vi "总氮流程.vi"   [LabVIEW 2016]
types:
  T1 = enum16{"步骤1", "步骤2", "步骤3", "步骤4", "步骤5", "步骤6", "步骤7", "步骤8", "步骤9", "步骤10"}
  T2 = enum32{"Bad", "Idle", "Run top level", "Running"}
  T3 = cluster{"系统时间":timestamp, "工作状态":u16, "测量模式":u16, "告警代码":enum16{"无告警", "缺试剂告警", "缺水样告警", "缺蒸馏水告警", "缺标液告警", "仪表漏液告警", "标定异常告警", "超量程告警", "加热异常", "低试剂预警", "超上限告警", "超下限告警", "仪表内部其他异常", "滴定异常告警", "电极异常告警", "量程切换告警", "参数设置告警", "PH电极电位异常", "电导率电极异常", "浊度光度异常", "溶解氧电极异常", "溶解氧光强异常", "温度异常告警", "PH异常告警", "溶解氧异常告警", "电导率异常告警", "浊度异常告警", "叶绿素异常告警", "藻密度异常告警", "蓝绿藻异常告警", "ORP异常告警", "氨氮异常告警", "清洁刷异常告警", "SD卡异常告警", "蓝牙异常告警", "Wifi异常告警", "流程异常告警"}, "故障代码":enum16{"无故障", "电机故障", "温度故障", "通讯故障", "滴定故障"}, "日志代码":u16, "软件版本":u16, "F0":sgl, "F1":sgl, "F2":sgl, "F3":sgl, "T":sgl, "H":sgl, "id":u16, "flowid":u16, "量程":u16}
  T4 = cluster{"因子编码":u32, "单位":u16, "标样参考值":sgl, "水样数据时间":timestamp, "水样实测值":sgl, "水样数据标识":string, "标样数据时间":timestamp, "标样实测值":sgl, "标样数据标识":string, "空白数据时间":timestamp, "空白实测值":sgl, "空白数据标识":string, "零点核查数据时间":timestamp, "零点核查实测值":sgl, "零点核查数据标识":string, "跨度核查数据时间":timestamp, "跨度核查实测值":sgl, "跨度核查数据标识":string, "加标回收数据时间":timestamp, "加标回收实测值":sgl, "加标回收数据标识":string, "平行样数据时间":timestamp, "平行样实测值":sgl, "平行样数据标识":string}
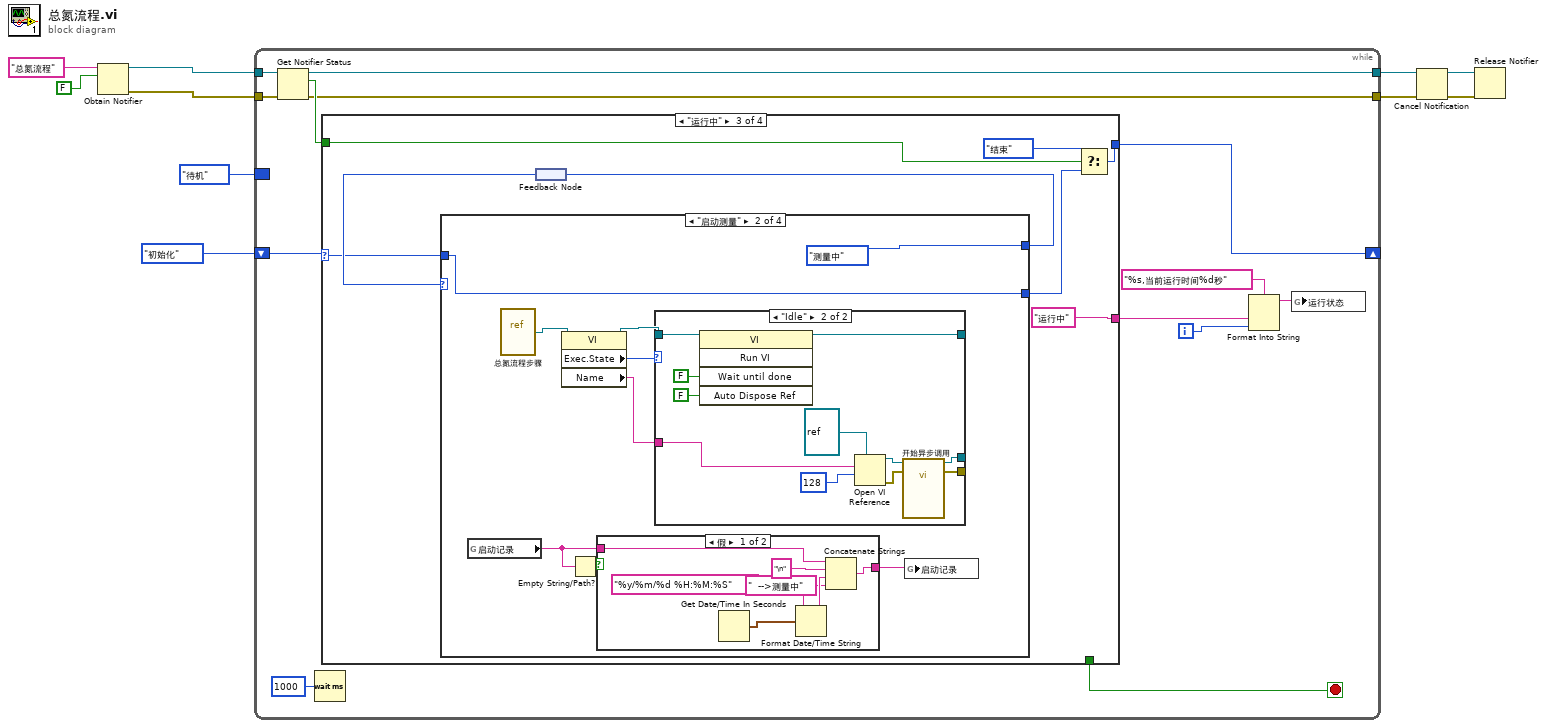
[diagram p0: block diagram]
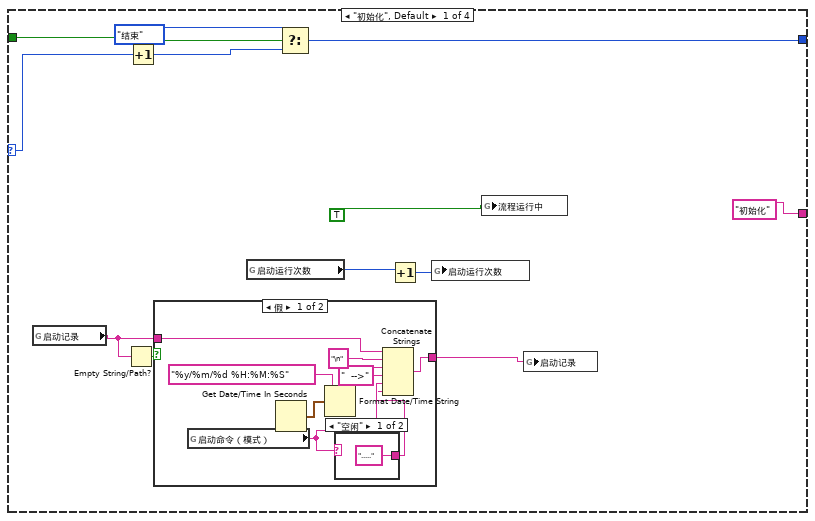
[diagram p2: hidden frame]
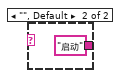
[diagram p3: hidden frame]
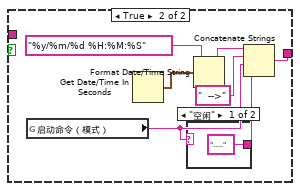
[diagram p4: hidden frame]
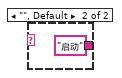
[diagram p5: hidden frame]
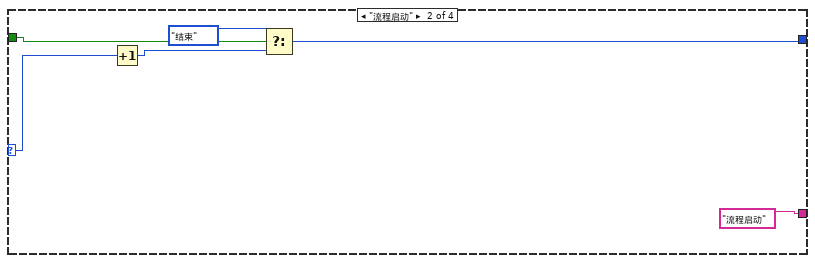
[diagram p6: hidden frame]
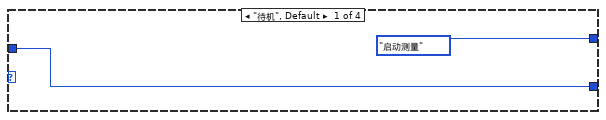
[diagram p7: hidden frame]
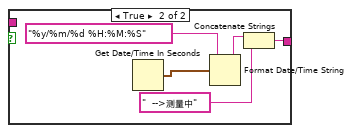
[diagram p8: hidden frame]
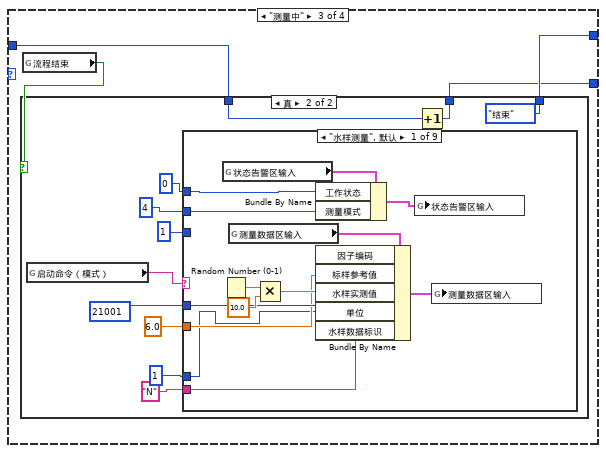
[diagram p10: hidden frame]
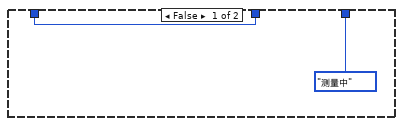
[diagram p11: hidden frame]
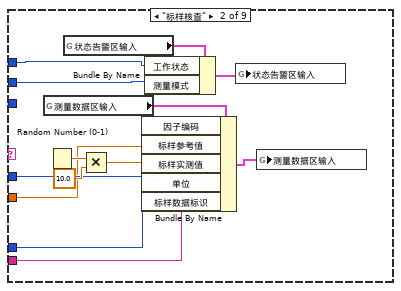
[diagram p12: hidden frame]
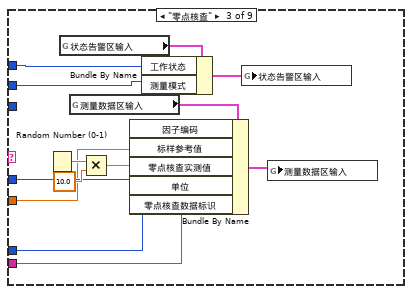
[diagram p13: hidden frame]
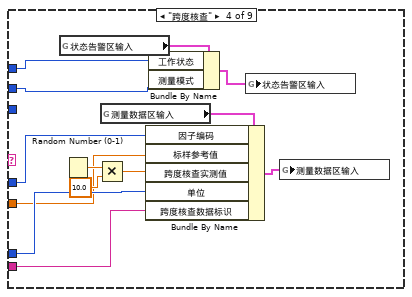
[diagram p14: hidden frame]
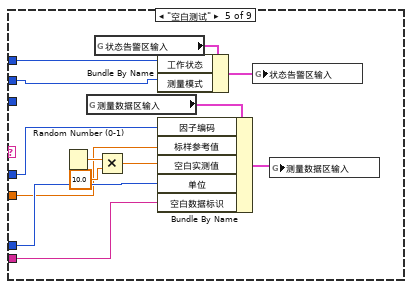
[diagram p15: hidden frame]
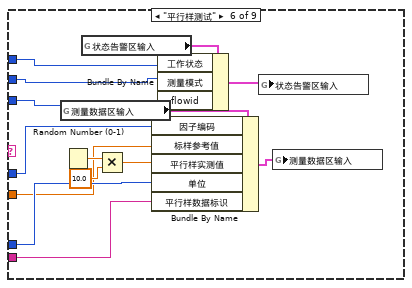
[diagram p16: hidden frame]
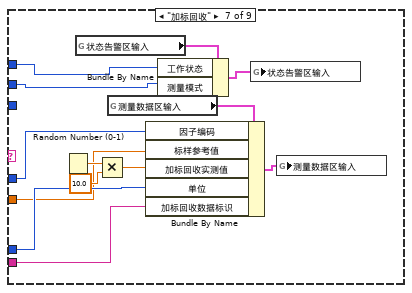
[diagram p17: hidden frame]
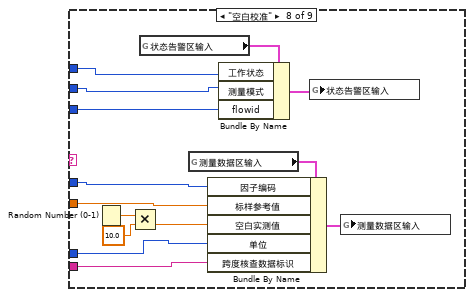
[diagram p18: hidden frame]
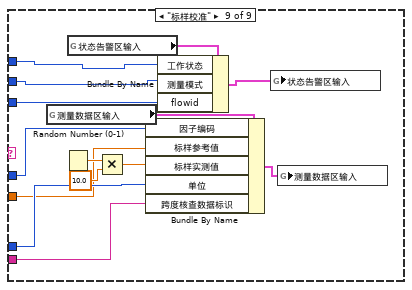
[diagram p19: hidden frame]
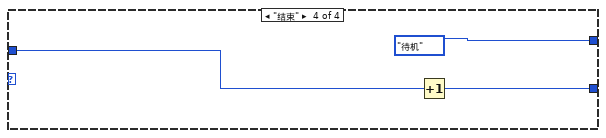
[diagram p20: hidden frame]
diagram:
  n1 = Obtain Notifier(name (unnamed)="总氮流程" ("名称（未命名）"), notification data type=FALSE) -> (notifier out=w7:refnum<notifier>, error out=w6:errorcluster)  [unwired: 2 in, 1 out]
  n2 = while {
    shift-right: [w20] -> _
    shift-left: enum16{"初始化", "流程启动", "运行中", "结束"}."初始化" ("枚举") -> [w23]
    tunnel: w7 -> [w15]
    tunnel: w6 -> [w14]
    tunnel: [w13] -> w5
    tunnel: [w12] -> w4
    border: enum16{"待机", "启动测量", "测量中", "结束"}."待机" -> [_]
    i -> [w18]
    stop <- w16 stop-if-true
    n3 = Get Notifier Status(notifier=w15, error in (no error)=w14) -> (notifier out=w13:refnum<notifier>, current notification=w21:bool, error out=w12:errorcluster)  [unwired: 2 out]
    n4 = Wait (ms)(milliseconds to wait=u32 1000 ("等待时间（毫秒）")) -> ()  [unwired: 1 out]
    n5 = case shown="\"运行中\"" w23 {
      selector: w23 -> [w33 w58 w64 w251]
      tunnel: [_ _ _ TRUE ("x")] -> w16
      tunnel: w21 -> [w35 w59 w68 _]
      tunnel: [w31 w57 w63 w251] -> w20
      tunnel: ["初始化" ("输入 1") "流程启动" ("输入 1") "运行中" ("输入 1") "结束" ("输入 1")] -> w17
      frame "初始化", Default {
        n6 = global read "总氮全局.vi" "启动记录"() -> (w25:string)
        n7 = Empty String/Path?(string/path=w25) -> (empty?=w29:bool)
        n8 = Increment(x=w33) -> (x+1=w32:enum16{"初始化", "流程启动", "运行中", "结束"})
        n9 = case shown="假" w29 {
          tunnel: w25 -> [w44 _]
          tunnel: [w39 w50] -> w24
          frame False {
            n10 = global read "总氮全局.vi" "启动命令（模式）"() -> (w37:string)
            n11 = Get Date/Time In Seconds() -> (seconds since 1Jan1904=w42:timestamp)
            n12 = Format Date/Time String(time format string (%c)="%y/%m/%d %H:%M:%S" ("时间格式字符串(%c)"), seconds (now)=w42) -> (date/time string=w40:string)  [unwired: 1 in]
            n13 = case shown="\"空闲\"" w37 {
              tunnel: ["....." ("字符串") "启动" ("字符串")] -> w36
              frame "空闲" {
              }
              frame "", Default {
              }
            }
            n14 = Concatenate Strings(w44, "\n" ("字符串"), w40, "  -->" ("字符串"), w37, w36) -> (w39:string)
          }
          frame True {
            n15 = global read "总氮全局.vi" "启动命令（模式）"() -> (w47:string)
            n16 = Get Date/Time In Seconds() -> (seconds since 1Jan1904=w53:timestamp)
            n17 = case shown="\"空闲\"" w47 {
              tunnel: ["....." ("字符串") "启动" ("字符串")] -> w48
              frame "空闲" {
              }
              frame "", Default {
              }
            }
            n18 = Format Date/Time String(time format string (%c)="%y/%m/%d %H:%M:%S" ("时间格式字符串(%c)"), seconds (now)=w53) -> (date/time string=w51:string)  [unwired: 1 in]
            n19 = Concatenate Strings(w51, "  -->" ("字符串"), w47, w48) -> (w50:string)
          }
        }
        n20 = global read "总氮全局.vi" "启动运行次数"() -> (w26:i32)
        n21 = Select(t=enum16{"初始化", "流程启动", "运行中", "结束"}."结束" ("枚举"), s=w35, f=w32) -> (s? t:f=w31:enum16{"初始化", "流程启动", "运行中", "结束"})
        n22 = Increment(x=w26) -> (x+1=w27:i32)
        n23 = global write "总氮全局.vi" "启动运行次数"(w27) -> ()
        n24 = global write "总氮全局.vi" "流程运行中"(TRUE ("流程运行中")) -> ()
        n25 = global write "总氮全局.vi" "启动记录"(w24) -> ()
      }
      frame "流程启动" {
        n26 = Increment(x=w58) -> (x+1=w60:enum16{"初始化", "流程启动", "运行中", "结束"})
        n27 = Select(t=enum16{"初始化", "流程启动", "运行中", "结束"}."结束" ("枚举"), s=w59, f=w60) -> (s? t:f=w57:enum16{"初始化", "流程启动", "运行中", "结束"})
      }
      frame "运行中" {
        n28 = feedback #1() -> (w67:enum16{"待机", "启动测量", "测量中", "结束"})
        n29 = case shown="\"启动测量\"" w67 {
          tunnel: [enum16{"待机", "启动测量", "测量中", "结束"}."启动测量" enum16{"待机", "启动测量", "测量中", "结束"}."测量中" w108 enum16{"待机", "启动测量", "测量中", "结束"}."待机"] -> w66
          tunnel: [w70 w79 w106 w243] -> w65
          tunnel: w64 -> [w70 w79 w107 w242]
          frame "待机", Default {
          }
          frame "启动测量" {
            n30 = global read "总氮全局.vi" "启动记录"() -> (w73:string)
            n31 = vi-ref "总氮流程步骤.vi"() -> (w75:refnum<vi>)
            n32 = property class="VI"(reference=w75) -> (reference out=w76:refnum<vi>, "Exec.State"=w77:T2, "Name"=w78:string)  [unwired: 1 in, 1 out]
            n33 = Empty String/Path?(string/path=w73) -> (empty?=w74:bool)
            n34 = case shown="假" w74 {
              tunnel: w73 -> [w87 _]
              tunnel: [w81 w88] -> w72
              frame False {
                n35 = Get Date/Time In Seconds() -> (seconds since 1Jan1904=w85:timestamp)
                n36 = Format Date/Time String(time format string (%c)="%y/%m/%d %H:%M:%S" ("时间格式字符串(%c)"), seconds (now)=w85) -> (date/time string=w83:string)  [unwired: 1 in]
                n37 = Concatenate Strings(w87, "\n" ("字符串"), w83, "  -->测量中" ("字符串")) -> (w81:string)
              }
              frame True {
                n38 = Get Date/Time In Seconds() -> (seconds since 1Jan1904=w92:timestamp)
                n39 = Format Date/Time String(time format string (%c)="%y/%m/%d %H:%M:%S" ("时间格式字符串(%c)"), seconds (now)=w92) -> (date/time string=w90:string)  [unwired: 1 in]
                n40 = Concatenate Strings(w90, "  -->测量中" ("字符串")) -> (w88:string)
              }
            }
            n41 = case shown="\"Idle\"" w77 {
              tunnel: w76 -> [w93 w101]
              tunnel: [w93 w102] -> _
              tunnel: w78 -> [_ w100]
              tunnel: [_ w95] -> _
              tunnel: [_ w94] -> _
              frame "Bad", Default {
              }
              frame "Idle" {
                n42 = invoke class="VI" method="Run VI"(reference=w101, "Wait until done"=FALSE ("结束前等待"), "Auto Dispose Ref"=FALSE ("自动销毁引用")) -> (reference out=w102:refnum<vi>)  [unwired: 2 in, 4 out]
                n43 = Open VI Reference(type specifier VI Refnum (for type only)=refnum<vi> refnum ("类型说明符VI引用句柄（仅用于类型）"), vi path=w100, options=128 ("选项")) -> (vi reference=w96:refnum<vi>, error out=w98:errorcluster)  [unwired: 3 in]
                n44 = call-by-ref "开始异步调用"(reference=w96, error in=w98) -> (reference out=w95:refnum<vi>, error out=w94:errorcluster)  [unwired: 12 in]
              }
            }
            n45 = global write "总氮全局.vi" "启动记录"(w72) -> ()
          }
          frame "测量中" {
            n46 = global read "总氮全局.vi" "流程结束"() -> (w105:bool)
            n47 = case shown="真" w105 {
              tunnel: [enum16{"待机", "启动测量", "测量中", "结束"}."测量中" enum16{"待机", "启动测量", "测量中", "结束"}."结束"] -> w108
              tunnel: w107 -> [w109 w114]
              tunnel: [w109 w113] -> w106
              frame False {
              }
              frame True {
                n48 = global read "总氮全局.vi" "启动命令（模式）"() -> (w111:string)
                n49 = case shown="\"水样测量\", 默认" w111 {
                  tunnel: u32 21001 ("因子编码") -> [w129 w144 w157 w169 w182 w196 w209 w223 w237]
                  tunnel: u16 4 ("测量模式") -> [w130 w143 w156 w170 w183 w197 w210 w224 w238]
                  tunnel: sgl 6.0 ("标样参考值") -> [w128 w142 w155 w167 w180 w194 w207 w221 w235]
                  tunnel: u16 1 ("单位") -> [w127 w141 w154 w168 w181 w195 w208 w222 w236]
                  tunnel: "N" -> [w131 w140 w153 w166 w179 w193 w206 w220 w234]
                  tunnel: u16 0 ("工作状态") -> [w126 w139 w152 w165 w178 w192 w205 w219 w233]
                  tunnel: u16 1 ("工作状态") -> [_ _ _ _ _ w191 _ w218 w232]
                  frame "水样测量", Default {
                    n50 = Random Number (0-1)() -> (number: 0 to 1=w132:dbl)
                    n51 = global read "总氮全局.vi" "状态告警区输入"() -> (w124:T3)
                    n52 = global read "总氮全局.vi" "测量数据区输入"() -> (w122:T4)
                    n53 = Multiply(x=w132, y=10.0 ("数字(0-1)")) -> (x*y=w134:dbl)
                    n54 = Bundle By Name(cluster=w124, "工作状态"=w126, "测量模式"=w130) -> (w125:T3)
                    n55 = Bundle By Name(cluster=w122, "因子编码"=w129, "标样参考值"=w128, "水样实测值"=w134, "单位"=w127, "水样数据标识"=w131) -> (w123:T4)
                    n56 = global write "总氮全局.vi" "状态告警区输入"(w125) -> ()
                    n57 = global write "总氮全局.vi" "测量数据区输入"(w123) -> ()
                  }
                  frame "标样核查" {
                    n58 = global read "总氮全局.vi" "测量数据区输入"() -> (w136:T4)
                    n59 = Random Number (0-1)() -> (number: 0 to 1=w145:dbl)
                    n60 = global read "总氮全局.vi" "状态告警区输入"() -> (w138:T3)
                    n61 = Multiply(x=w145, y=10.0 ("数字(0-1)")) -> (x*y=w147:dbl)
                    n62 = Bundle By Name(cluster=w136, "因子编码"=w144, "标样参考值"=w142, "标样实测值"=w147, "单位"=w141, "标样数据标识"=w140) -> (w135:T4)
                    n63 = Bundle By Name(cluster=w138, "工作状态"=w139, "测量模式"=w143) -> (w137:T3)
                    n64 = global write "总氮全局.vi" "状态告警区输入"(w137) -> ()
                    n65 = global write "总氮全局.vi" "测量数据区输入"(w135) -> ()
                  }
                  frame "零点核查" {
                    n66 = Random Number (0-1)() -> (number: 0 to 1=w158:dbl)
                    n67 = global read "总氮全局.vi" "状态告警区输入"() -> (w151:T3)
                    n68 = global read "总氮全局.vi" "测量数据区输入"() -> (w149:T4)
                    n69 = Multiply(x=w158, y=10.0 ("数字(0-1)")) -> (x*y=w160:dbl)
                    n70 = Bundle By Name(cluster=w149, "因子编码"=w157, "标样参考值"=w155, "零点核查实测值"=w160, "单位"=w154, "零点核查数据标识"=w153) -> (w148:T4)
                    n71 = Bundle By Name(cluster=w151, "工作状态"=w152, "测量模式"=w156) -> (w150:T3)
                    n72 = global write "总氮全局.vi" "状态告警区输入"(w150) -> ()
                    n73 = global write "总氮全局.vi" "测量数据区输入"(w148) -> ()
                  }
                  frame "跨度核查" {
                    n74 = global read "总氮全局.vi" "状态告警区输入"() -> (w162:T3)
                    n75 = Random Number (0-1)() -> (number: 0 to 1=w171:dbl)
                    n76 = Multiply(x=w171, y=10.0 ("数字(0-1)")) -> (x*y=w173:dbl)
                    n77 = global read "总氮全局.vi" "测量数据区输入"() -> (w164:T4)
                    n78 = Bundle By Name(cluster=w164, "因子编码"=w169, "标样参考值"=w167, "跨度核查实测值"=w173, "单位"=w168, "跨度核查数据标识"=w166) -> (w163:T4)
                    n79 = Bundle By Name(cluster=w162, "工作状态"=w165, "测量模式"=w170) -> (w161:T3)
                    n80 = global write "总氮全局.vi" "状态告警区输入"(w161) -> ()
                    n81 = global write "总氮全局.vi" "测量数据区输入"(w163) -> ()
                  }
                  frame "空白测试" {
                    n82 = Random Number (0-1)() -> (number: 0 to 1=w184:dbl)
                    n83 = global read "总氮全局.vi" "测量数据区输入"() -> (w175:T4)
                    n84 = global read "总氮全局.vi" "状态告警区输入"() -> (w177:T3)
                    n85 = Multiply(x=w184, y=10.0 ("数字(0-1)")) -> (x*y=w186:dbl)
                    n86 = Bundle By Name(cluster=w177, "工作状态"=w178, "测量模式"=w183) -> (w176:T3)
                    n87 = Bundle By Name(cluster=w175, "因子编码"=w182, "标样参考值"=w180, "空白实测值"=w186, "单位"=w181, "空白数据标识"=w179) -> (w174:T4)
                    n88 = global write "总氮全局.vi" "状态告警区输入"(w176) -> ()
                    n89 = global write "总氮全局.vi" "测量数据区输入"(w174) -> ()
                  }
                  frame "平行样测试" {
                    n90 = global read "总氮全局.vi" "测量数据区输入"() -> (w190:T4)
                    n91 = Random Number (0-1)() -> (number: 0 to 1=w198:dbl)
                    n92 = global read "总氮全局.vi" "状态告警区输入"() -> (w188:T3)
                    n93 = Multiply(x=w198, y=10.0 ("数字(0-1)")) -> (x*y=w200:dbl)
                    n94 = Bundle By Name(cluster=w190, "因子编码"=w196, "标样参考值"=w194, "平行样实测值"=w200, "单位"=w195, "平行样数据标识"=w193) -> (w189:T4)
                    n95 = Bundle By Name(cluster=w188, "工作状态"=w192, "测量模式"=w197, "flowid"=w191) -> (w187:T3)
                    n96 = global write "总氮全局.vi" "状态告警区输入"(w187) -> ()
                    n97 = global write "总氮全局.vi" "测量数据区输入"(w189) -> ()
                  }
                  frame "加标回收" {
                    n98 = Random Number (0-1)() -> (number: 0 to 1=w211:dbl)
                    n99 = global read "总氮全局.vi" "状态告警区输入"() -> (w201:T3)
                    n100 = Multiply(x=w211, y=10.0 ("数字(0-1)")) -> (x*y=w213:dbl)
                    n101 = global read "总氮全局.vi" "测量数据区输入"() -> (w204:T4)
                    n102 = Bundle By Name(cluster=w204, "因子编码"=w209, "标样参考值"=w207, "加标回收实测值"=w213, "单位"=w208, "加标回收数据标识"=w206) -> (w203:T4)
                    n103 = Bundle By Name(cluster=w201, "工作状态"=w205, "测量模式"=w210) -> (w202:T3)
                    n104 = global write "总氮全局.vi" "状态告警区输入"(w202) -> ()
                    n105 = global write "总氮全局.vi" "测量数据区输入"(w203) -> ()
                  }
                  frame "空白校准" {
                    n106 = Random Number (0-1)() -> (number: 0 to 1=w225:dbl)
                    n107 = Multiply(x=w225, y=10.0 ("数字(0-1)")) -> (x*y=w227:dbl)
                    n108 = global read "总氮全局.vi" "状态告警区输入"() -> (w215:T3)
                    n109 = global read "总氮全局.vi" "测量数据区输入"() -> (w217:T4)
                    n110 = Bundle By Name(cluster=w217, "因子编码"=w223, "标样参考值"=w221, "空白实测值"=w227, "单位"=w222, "跨度核查数据标识"=w220) -> (w216:T4)
                    n111 = Bundle By Name(cluster=w215, "工作状态"=w219, "测量模式"=w224, "flowid"=w218) -> (w214:T3)
                    n112 = global write "总氮全局.vi" "状态告警区输入"(w214) -> ()
                    n113 = global write "总氮全局.vi" "测量数据区输入"(w216) -> ()
                  }
                  frame "标样校准" {
                    n114 = global read "总氮全局.vi" "测量数据区输入"() -> (w231:T4)
                    n115 = Random Number (0-1)() -> (number: 0 to 1=w239:dbl)
                    n116 = global read "总氮全局.vi" "状态告警区输入"() -> (w228:T3)
                    n117 = Multiply(x=w239, y=10.0 ("数字(0-1)")) -> (x*y=w241:dbl)
                    n118 = Bundle By Name(cluster=w231, "因子编码"=w237, "标样参考值"=w235, "标样实测值"=w241, "单位"=w236, "跨度核查数据标识"=w234) -> (w230:T4)
                    n119 = Bundle By Name(cluster=w228, "工作状态"=w233, "测量模式"=w238, "flowid"=w232) -> (w229:T3)
                    n120 = global write "总氮全局.vi" "状态告警区输入"(w229) -> ()
                    n121 = global write "总氮全局.vi" "测量数据区输入"(w230) -> ()
                  }
                }
                n122 = Increment(x=w114) -> (x+1=w113:enum16{"初始化", "流程启动", "运行中", "结束"})
              }
            }
          }
          frame "结束" {
            n123 = Increment(x=w242) -> (x+1=w243:enum16{"初始化", "流程启动", "运行中", "结束"})
          }
        }
        n124 = feedback-in #1(w66) -> ()
        n125 = Select(t=enum16{"初始化", "流程启动", "运行中", "结束"}."结束" ("枚举"), s=w68, f=w65) -> (s? t:f=w63:enum16{"初始化", "流程启动", "运行中", "结束"})
      }
      frame "结束" {
        w247 = FALSE ("流程结束")
        # "流程结束"
        n126 = global read "总氮全局.vi" "启动记录"() -> (w249:string)
        n127 = Empty String/Path?(string/path=w249) -> (empty?=w250:bool)
        n128 = case shown="真" w250 {
          tunnel: w249 -> [w260 _]
          tunnel: [w254 w261] -> w248
          frame False {
            n129 = Get Date/Time In Seconds() -> (seconds since 1Jan1904=w258:timestamp)
            n130 = Format Date/Time String(time format string (%c)="%y/%m/%d %H:%M:%S" ("时间格式字符串(%c)"), seconds (now)=w258) -> (date/time string=w256:string)  [unwired: 1 in]
            n131 = Concatenate Strings(w260, "\n" ("字符串"), w256, "  -->结束" ("字符串")) -> (w254:string)
          }
          frame True {
            n132 = Get Date/Time In Seconds() -> (seconds since 1Jan1904=w265:timestamp)
            n133 = Format Date/Time String(time format string (%c)="%y/%m/%d %H:%M:%S" ("时间格式字符串(%c)"), seconds (now)=w265) -> (date/time string=w263:string)  [unwired: 1 in]
            n134 = Concatenate Strings(w263, "  -->结束" ("字符串")) -> (w261:string)
          }
        }
        n135 = global write "总氮全局.vi" "启动记录"(w248) -> ()
        n136 = global write "总氮全局.vi" "步骤运行时间/秒"(0 ("运行时间/秒")) -> ()
        n137 = global write "总氮全局.vi" "流程结束"(w247) -> ()
        n138 = global write "总氮全局.vi" "流程运行中"(w247) -> ()
        n139 = global write "总氮全局.vi" "当前步骤"(T1."步骤1" ("当前步骤 2")) -> ()
      }
    }
    n140 = Format Into String(format string="%s,当前运行时间%d秒" ("格式字符串"), w17, w18) -> (resulting string=w11:string)  [unwired: 2 in, 1 out]
    n141 = global write "总氮全局.vi" "运行状态"(w11) -> ()
  }
  n142 = Cancel Notification(0:w5, 3:w4) -> (8:w3:refnum<notifier>, 11:w2:errorcluster)  [unwired: 1 out]
  n143 = Release Notifier(notifier=w3, error in (no error)=w2) -> ()  [unwired: 1 in, 3 out]
